vi "Close Hardware.vi"(8 "error in (no error)":errorcluster, 11 "Application in":refnum<class "Application.lvclass">) -> (0 "error out":errorcluster, 3 "Application out":refnum<class "Application.lvclass">)   [LabVIEW 2017, in "Application.lvlib" / "Application.lvclass"]
uses:
  Application.lvclass
  Instruments/Instrument/Class/Instrument.lvclass
  C:/Program Files (x86)/National Instruments/LabVIEW 2017/vi.lib/TSS/ACRObat Test Framework/Classes/Base Objects/Base Class/Base Class/Base Class.lvclass
  <vilib>/TSS/ACRObat Test Framework/Classes/Base Objects/Base Class/Base Class/Base Class.lvclass
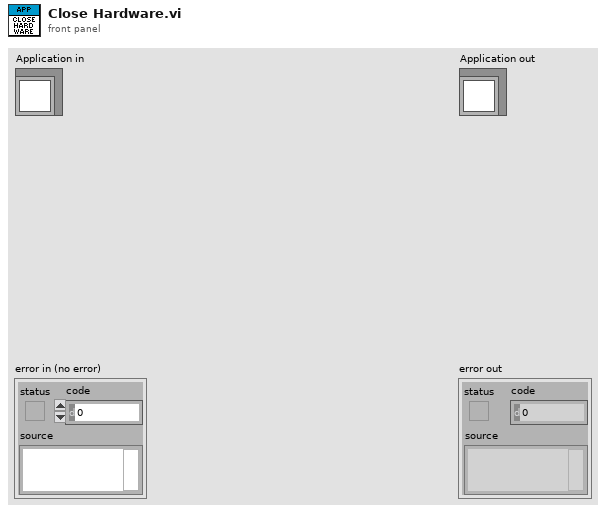
[diagram p1: front panel]
types:
  T1 = typedef "Application.lvlib/App Properties.lvclass/Class Properties -- Cluster.ctl" = cluster{"UUT Info":T2[], "Test Information":refnum<vi>, "Gold Board":refnum<class "Golden Board.lvclass">, "Test Recipe":refnum<class "Test Recipe.lvclass">, "Instruments":refnum<class "Instrument.lvclass">[], "Mode":T3, "Test Results":T4[], "Station Config":refnum<class "Station Config.lvclass">, "Variable Engine":refnum<class "Variable Engine.lvclass">}
  T2 = typedef "Application.lvlib/App Properties.lvclass/UUT Reference -- Cluster.ctl" = cluster{"Serial Number Reference":refnum<vi>, "Status Message Reference":refnum<vi>}
  T3 = typedef "Application.lvlib/Application.lvclass/Op Mode -- Enum.ctl" = u16
  T4 = typedef "Application.lvlib/App Properties.lvclass/Test Result -- Cluster.ctl" = cluster{"Position":i32, "Pass":bool, "Fail Codes":string}
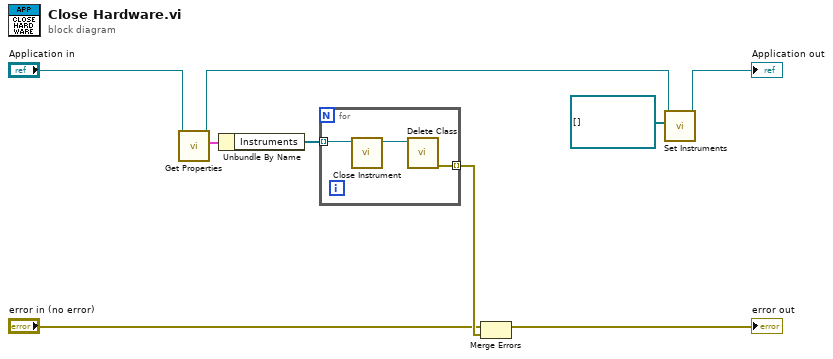
[diagram p0: block diagram]
diagram:
  n1 = call "Get Properties.vi"("Acrobat Template in"="Application in") -> ("Class Properties"=w7:T1, "Acrobat Template out"=w4:refnum<class "Application.lvclass">)  [unwired: 8 in, 1 out]
  n2 = Unbundle By Name(w7) -> ("Instruments"=w6:refnum<class "Instrument.lvclass">[])
  n3 = for {
    tunnel: w6 -> [w11] mode=indexing
    tunnel: [w12] -> w5 mode=indexing
    n4 = call-dynamic "Close Instrument.vi"("Instrument in"=w11) -> ("Instrument out"=w10:refnum<class "Instrument.lvclass">)  [unwired: 9 in, 1 out]
    n5 = call <vilib>:"Delete Class.vi"("Base Class in"=w10) -> ("error out"=w12:errorcluster)  [unwired: 9 in, 1 out]
  }
  n6 = Merge Errors("error in (no error)", w5) -> (→"error out":errorcluster)
  n7 = call "Set Instruments.vi"("Instruments"=refnum<class "Instrument.lvclass">[] [], "Acrobat Template in"=w4) -> ("Acrobat Template out"=→"Application out":refnum<class "Application.lvclass">)  [unwired: 8 in, 1 out]
